vi "Try Match Response.vi"(8 "error in":errorcluster, 10 "ICAN CC Frame":refnum<class "ICAN CC Frame.lvclass">, 11 "IResponse in":refnum<class "IMatch Response.lvclass">) -> (0 "error out":errorcluster, 2 "Match":bool, 3 "IResponse out":refnum<class "IMatch Response.lvclass">)   [LabVIEW 2020, in "CANopen.lvlib" / "IMatch Response.lvclass"]
uses:
  IMatch Response.lvclass
  HAL/Source/Interfaces/ICAN CC Frame/ICAN CC Frame.lvclass
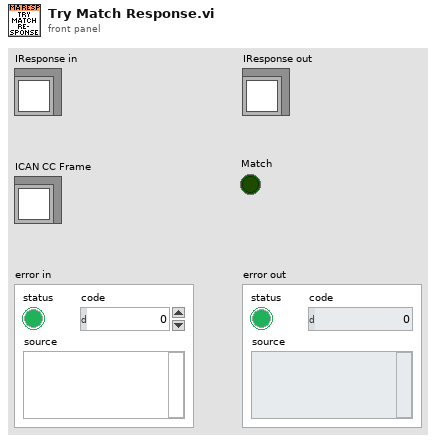
[diagram p1: front panel]
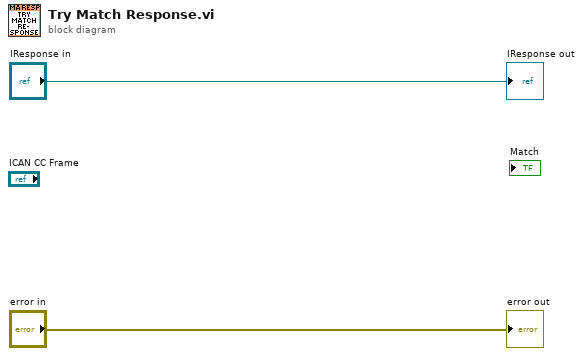
[diagram p0: block diagram]
diagram:
  "IResponse out" <- "IResponse in"
  "error out" <- "error in"
